vi "Add entry to combo box.vi"(4 "error in":errorcluster, 6 "Value":string, 7 "CmbBox Refnum":refnum<vi>) -> (0 "error out":errorcluster)   [LabVIEW 2014]
doc: "Add entry to combo box control."
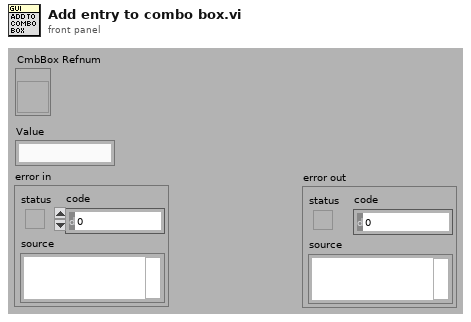
[diagram p1: front panel]
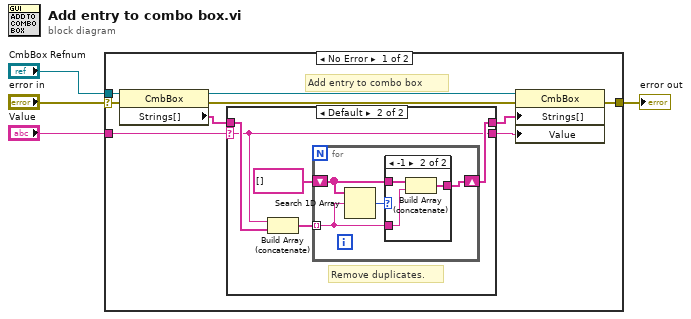
[diagram p0: block diagram]
diagram:
  n1 = case shown="No Error" "error in" {
    selector: "error in" -> [w5 w28]
    tunnel: [w11 w28] -> w4
    tunnel: "CmbBox Refnum" -> [w8 _]
    tunnel: "Value" -> [w7 _]
    frame No Error {
      # "Add entry to combo box"
      n2 = property on="Property Node" class="CmbBox"(reference=w8, error in=w5) -> (error out=w10:errorcluster, "Strings[]"=w9:string[])  [unwired: 1 out]
      n3 = case shown="Default" w7 {
        selector: w7 -> [w13 w15]
        tunnel: [w14 w19] -> w12
        tunnel: w9 -> [w14 w16]
        tunnel: [w13 w15] -> w6
        frame "" {
        }
        frame Default {
          # "Remove duplicates."
          n4 = Build Array (concatenate)(w15, w16) -> (w18:string[])
          n5 = for {
            tunnel: w18 -> [w22] mode=indexing
            shift-right: [w21] -> w19
            shift-left: string[] [] -> [w20]
            n6 = Search 1D Array(1D array=w20, element=w22) -> (index of element=w23:i32)  [unwired: 1 out]
            n7 = case shown="-1" w23 {
              tunnel: w22 -> [_ w27]
              tunnel: [w24 w25] -> w21
              tunnel: w20 -> [w24 w26]
              frame Default {
              }
              frame -1 {
                n8 = Build Array (concatenate)(w26, w27) -> (w25:string[])
              }
            }
          }
        }
      }
      n9 = property on="Property Node" class="CmbBox"(reference=w8, error in=w10, "Strings[]"=w12, "Value"=w6) -> (error out=w11:errorcluster)  [unwired: 1 out]
    }
    frame Error {
    }
  }
  "error out" <- w4
